vi "Obtain Notifier.vi"(8 "Error In":errorcluster, 11 "Name":string) -> (0 "Error Out":errorcluster, 3 "notifier out":refnum<notifier>)   [LabVIEW 2019, in "Error Notifier.lvlib"]
uses:
  Error Notifier.lvlib
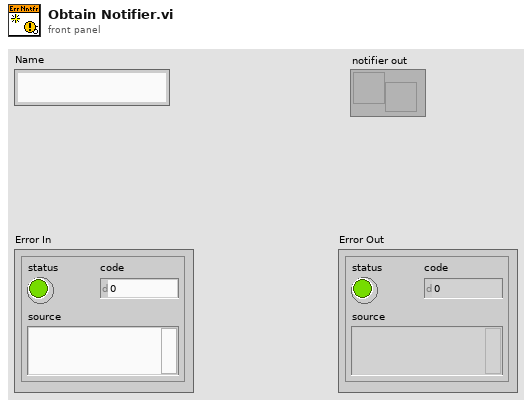
[diagram p1: front panel]
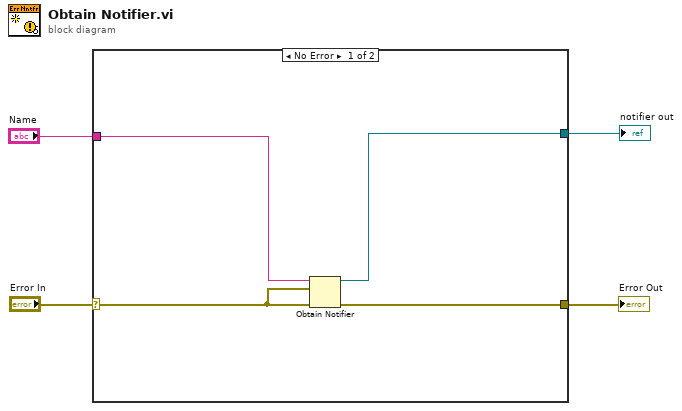
[diagram p0: block diagram]
diagram:
  n1 = case shown="No Error" "Error In" {
    selector: "Error In" -> [w7 w9]
    tunnel: [w8 w9] -> w3
    tunnel: "Name" -> [w6 _]
    tunnel: [w5 _] -> w1
    frame No Error {
      n2 = Obtain Notifier(name (unnamed)=w6, notification data type=w7, error in (no error)=w7) -> (notifier out=w5:refnum<notifier>, error out=w8:errorcluster)  [unwired: 1 in, 1 out]
    }
    frame Error {
    }
  }
  "Error Out" <- w3
  "notifier out" <- w1
